vi "CtrlAll.vi"(11 "SRE Enum":enum16{"Start", "Run", "End"}(ring)) -> ()   [LabVIEW 2014]
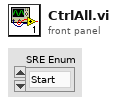
[diagram p1: front panel]
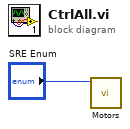
[diagram p0: block diagram]
diagram:
  n1 = call "Motors.vi"("SRE Enum"="SRE Enum") -> ()  [unwired: 11 in]
